vi "getDescription.vi"(8 "error in (no error)":errorcluster, 11 "Camera in":refnum<class "Camera.lvclass">) -> (0 "error out":errorcluster, 2 "description":T1={"serial"=4294967295, "type"=0, "sub_type"=0, "interface_type"=0, "bit_resolution"=0, "min_exposure_time_s"=nan, "max_exposure_time_s"=nan, "min_exposure_step_s"=nan, "min_delay_time_s"=nan, "max_delay_time_s"=nan, "min_delay_step_s"=nan, "min_width"=18446744073709551615, "min_height"=18446744073709551615, "max_width"=18446744073709551615, "max_height"=18446744073709551615, "roi_step_horz"=18446744073709551615, "roi_step_vert"=18446744073709551615, "roi_symmetric_horz"=FALSE, "roi_symmetric_vert"=FALSE, "has_timestamp_mode"=FALSE, "has_timestamp_mode_ascii_only"=FALSE, "pixelrate_vec"=[], "has_acquire_mode"=FALSE, "has_ext_acquire_mode"=FALSE, "has_metadata_mode"=FALSE, "has_ram"=FALSE, "binning_horz_vec"=[], "binning_vert_vec"=[]}, 3 "Camera out":refnum<class "Camera.lvclass">)   [LabVIEW 2020, in "Camera.lvclass"]
doc: "Gets the current configuration from the camera."
uses:
  Camera.lvclass
  Camera.lvclass/Camera.ctl
  CameraDescription.lvlib
  ImageSensor.lvlib
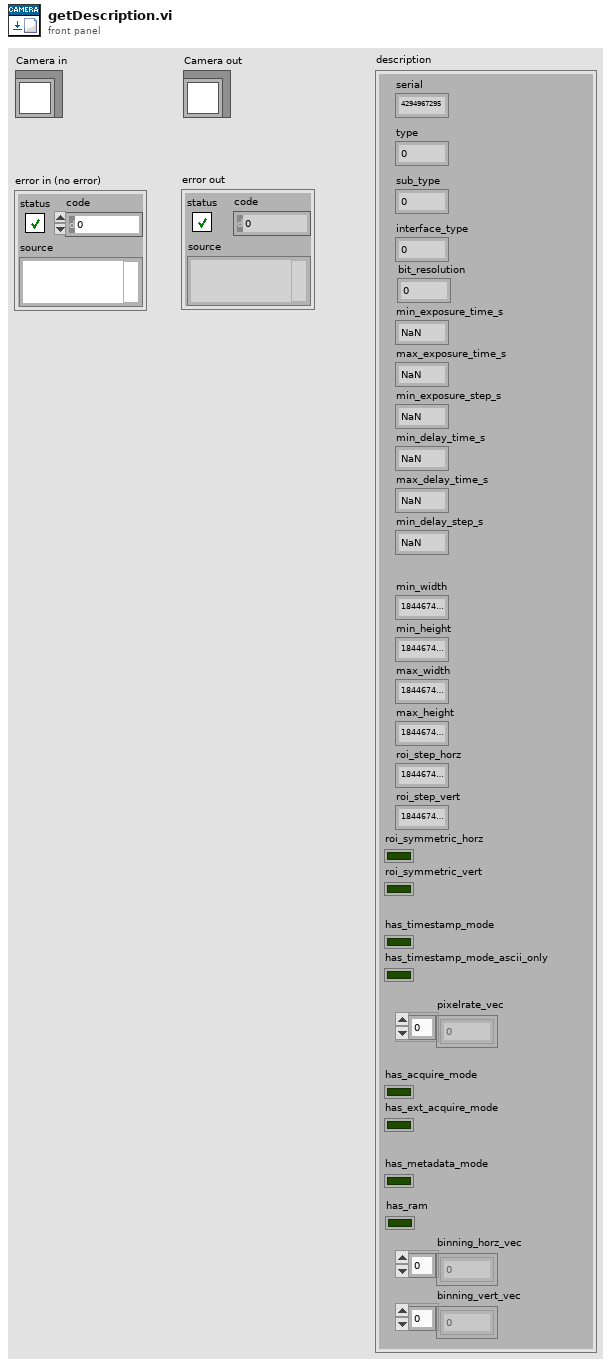
[diagram p1: front panel]
types:
  T1 = cluster{"serial":u32, "type":u16, "sub_type":u16, "interface_type":u16, "bit_resolution":u16, "min_exposure_time_s":dbl, "max_exposure_time_s":dbl, "min_exposure_step_s":dbl, "min_delay_time_s":dbl, "max_delay_time_s":dbl, "min_delay_step_s":dbl, "min_width":u64, "min_height":u64, "max_width":u64, "max_height":u64, "roi_step_horz":u64, "roi_step_vert":u64, "roi_symmetric_horz":bool, "roi_symmetric_vert":bool, "has_timestamp_mode":bool, "has_timestamp_mode_ascii_only":bool, "pixelrate_vec":u32[], "has_acquire_mode":bool, "has_ext_acquire_mode":bool, "has_metadata_mode":bool, "has_ram":bool, "binning_horz_vec":u16[], "binning_vert_vec":u16[]}
  T2 = cluster{"wSensorTypeDESC":u16, "wSensorSubTypeDESC":u16, "wMaxHorzResStdDESC":u16, "wMaxVertResStdDESC":u16, "wMaxHorzResExtDESC":u16, "wMaxVertResExtDESC":u16, "wDynResDESC":u16, "wMaxBinHorzDESC":u16, "wBinHorzSteppingDESC":u16, "wMaxBinVertDESC":u16, "wBinVertSteppingDESC":u16, "wRoiHorStepsDESC":u16, "wRoiVertStepsDESC":u16, "wNumADCsDESC":u16, "wMinSizeHorzDESC":u16, "dwPixelRateDESC":u32[], "wConvFactDESC":u16[], "sCoolingSetpoints":i16[], "wSoftRoiHorStepsDESC":u16, "wSoftRoiVertStepsDESC":u16, "wIRDESC":u16, "wMinSizeVertDESC":u16, "dwMinDelayDESC":u32, "dwMaxDelayDESC":u32, "dwMinDelayStepDESC":u32, "dwMinExposureDESC":u32, "dwMaxExposureDESC":u32, "dwMinExposureStepDESC":u32, "dwMinDelayIRDESC":u32, "dwMaxDelayIRDESC":u32, "dwMinExposureIRDESC":u32, "dwMaxExposureIRDESC":u32, "wTimeTableDESC":u16, "wDoubleImageDESC":u16, "sMinCoolSetDESC":i16, "sMaxCoolSetDESC":i16, "sDefaultCoolSetDESC":i16, "wPowerDownModeDESC":u16, "wOffsetRegulationDESC":u16, "wColorPatternDESC":u16, "wPatternTypeDESC":u16, "wNumCoolingSetpoints":u16, "dwGeneralCapsDESC1":u32, "dwGeneralCapsDESC2":u32, "dwExtSyncFrequency":u32[], "dwGeneralCapsDESC3":u32, "dwGeneralCapsDESC4":u32}
  T3 = cluster{"wDarkOffsetDESC3":u16, "dwGeneralCapsDESC3_1":u32, "dwGeneralCapsDESC3_2":u32, "dwGeneralCapsDESC3_3":u32, "dwGeneralCapsDESC3_4":u32, "wMinHorzResStdDESC3":u16, "wMinVertResStdDESC3":u16, "wMinHorzResExtDESC3":u16, "wMinVertResExtDESC3":u16, "dPixelsize_horzDESC3_um":dbl, "dPixelsize_vertDESC3_um":dbl, "dMinSensorTempWarningDESC3_C":dbl, "dMaxSensorTempWarningDESC3_C":dbl, "dMinCameraTempWarningDESC3_C":dbl, "dMaxCameraTempWarningDESC3_C":dbl, "dMinPowerTempWarningDESC3_C":dbl, "dMaxPowerTempWarningDESC3_C":dbl, "dMinPowerVoltageWarningDESC3_V":dbl, "dMaxPowerVoltageWarningDESC3_V":dbl, "dMinSensorTempErrorDESC3_C":dbl, "dMaxSensorTempErrorDESC3_C":dbl, "dMinCameraTempErrorDESC3_C":dbl, "dMaxCameraTempErrorDESC3_C":dbl, "dMinPowerTempErrorDESC3_C":dbl, "dMaxPowerTempErrorDESC3_C":dbl, "dMinPowerVoltageErrorDESC3_V":dbl, "dMaxPowerVoltageErrorDESC3_V":dbl}
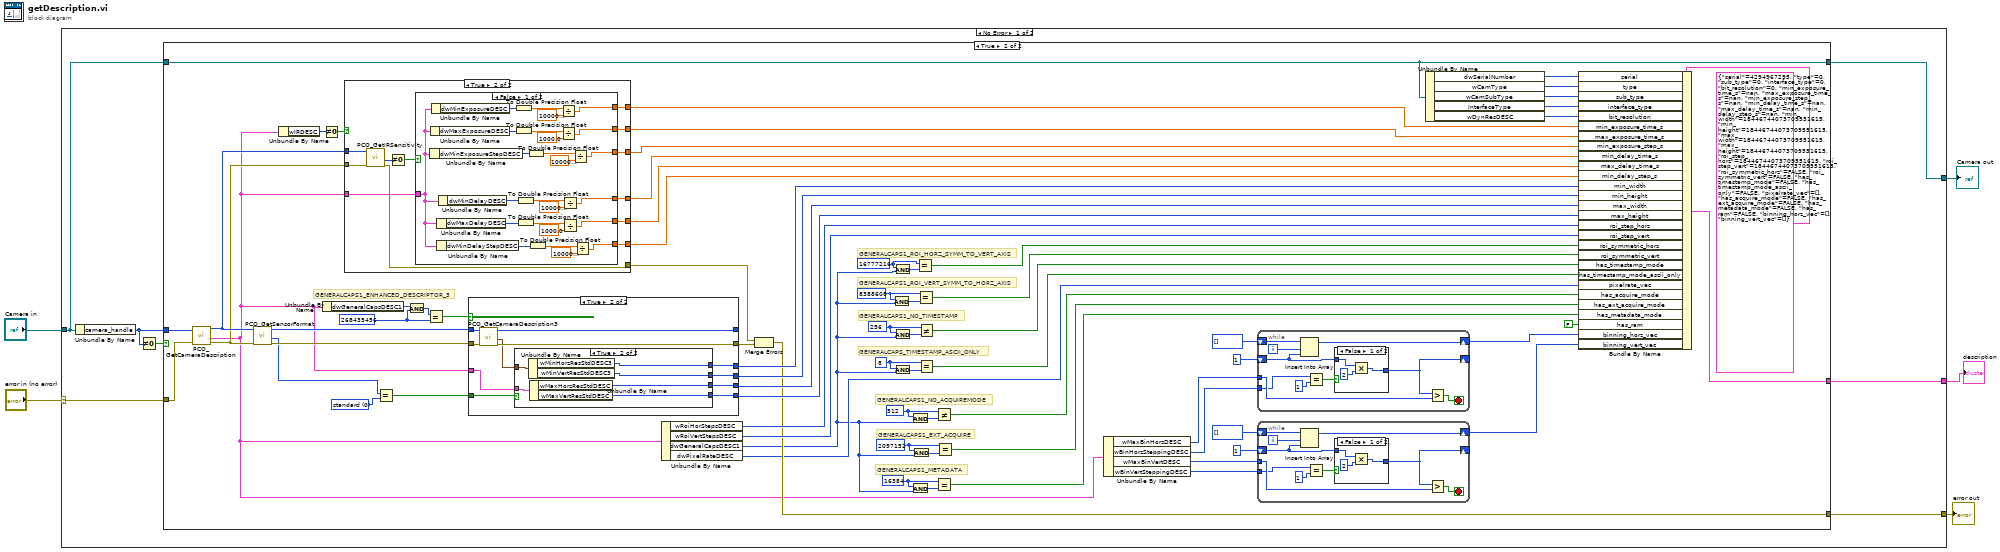
[diagram p0: block diagram]
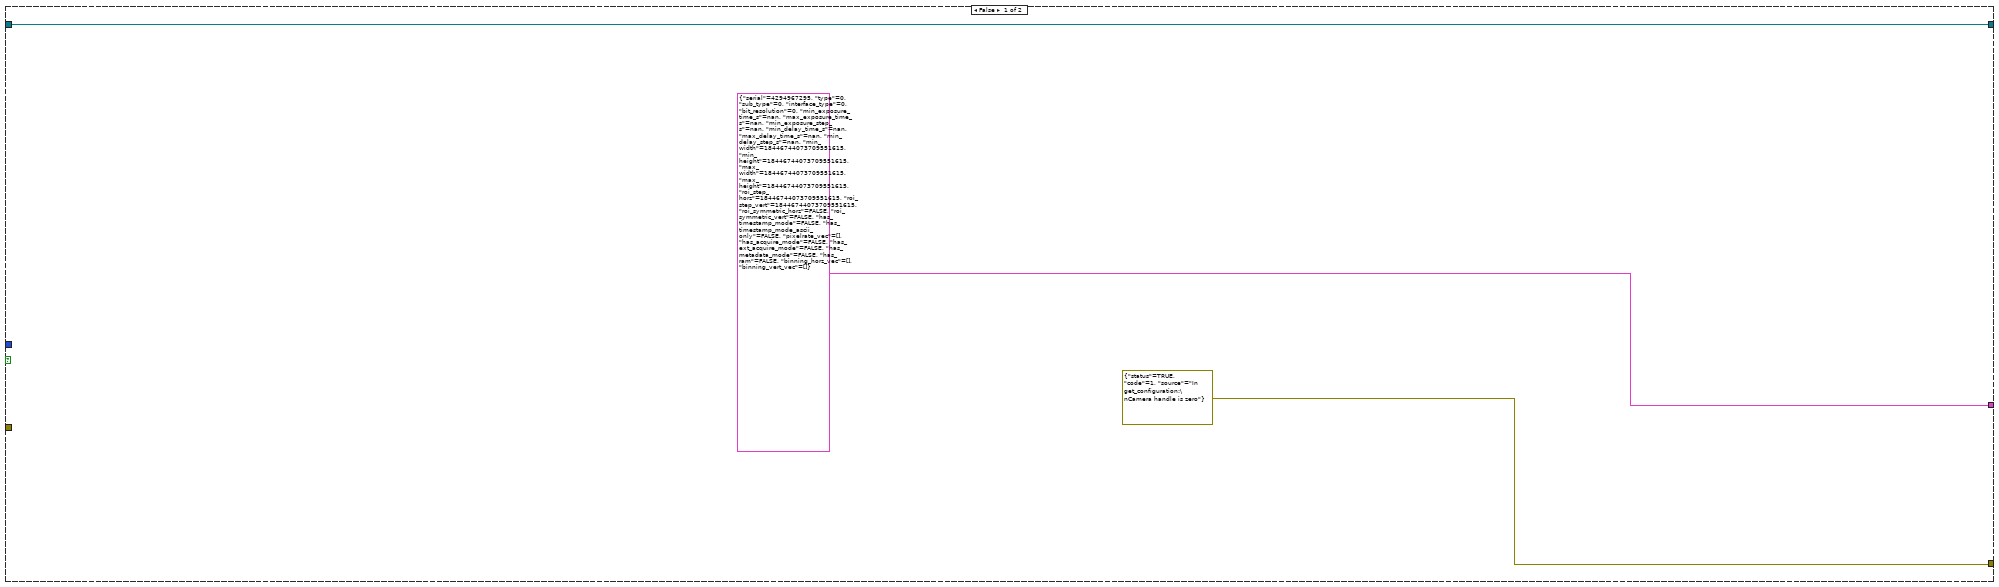
[diagram p2: hidden frame]
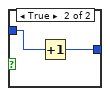
[diagram p3: hidden frame]
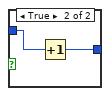
[diagram p4: hidden frame]
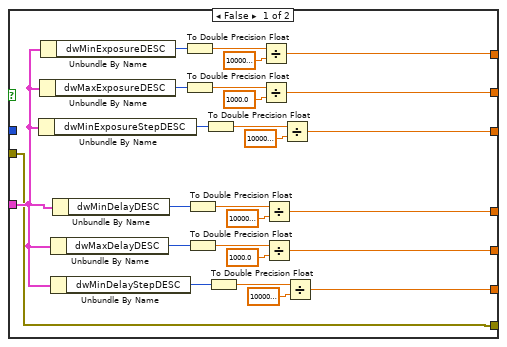
[diagram p5: hidden frame]
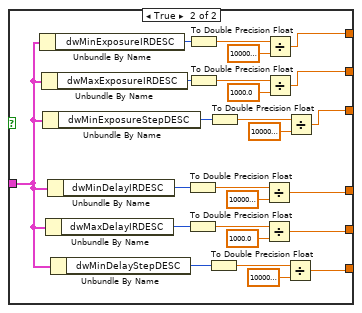
[diagram p6: hidden frame]
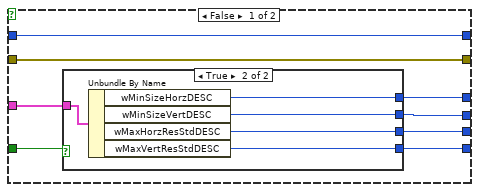
[diagram p7: hidden frame]
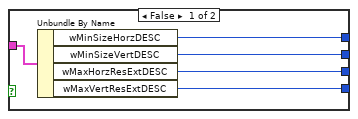
[diagram p8: hidden frame]
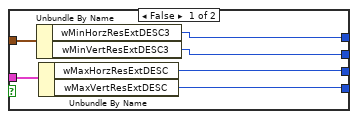
[diagram p9: hidden frame]
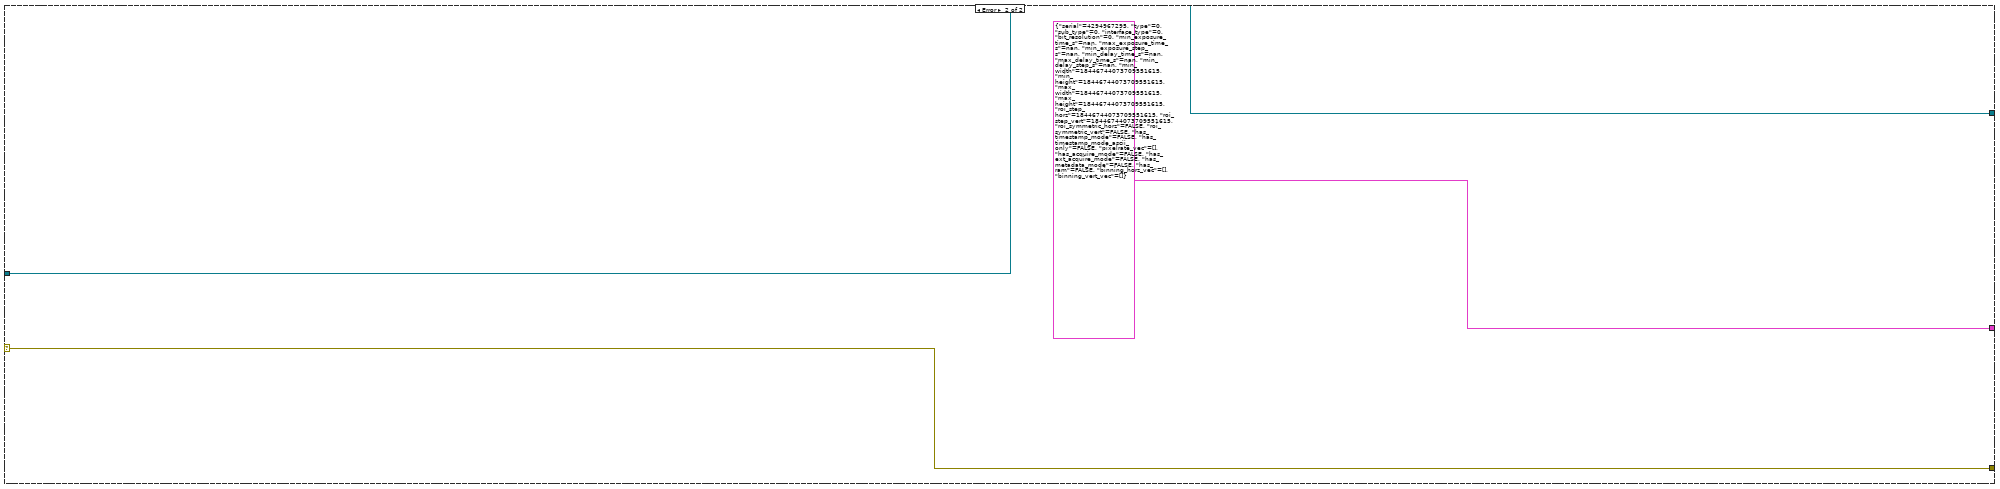
[diagram p10: hidden frame]
diagram:
  n1 = case shown="No Error" "error in (no error)" {
    selector: "error in (no error)" -> [w9 w250]
    tunnel: [w11 w250] -> w4
    tunnel: [w6 w249] -> w2
    tunnel: "Camera in" -> [w8 w249]
    tunnel: [w7 T1 {"serial"=4294967295, "type"=0, "sub_type"=0, "interface_type"=0, "bit_resolution"=0, "min_exposure_time_s"=nan, "max_exposure_time_s"=nan, "min_exposure_step_s"=nan, "min_delay_time_s"=nan, "max_delay_time_s"=nan, "min_delay_step_s"=nan, "min_width"=18446744073709551615, "min_height"=18446744073709551615, "max_width"=18446744073709551615, "max_height"=18446744073709551615, "roi_step_horz"=18446744073709551615, "roi_step_vert"=18446744073709551615, "roi_symmetric_horz"=FALSE, "roi_symmetric_vert"=FALSE, "has_timestamp_mode"=FALSE, "has_timestamp_mode_ascii_only"=FALSE, "pixelrate_vec"=[], "has_acquire_mode"=FALSE, "has_ext_acquire_mode"=FALSE, "has_metadata_mode"=FALSE, "has_ram"=FALSE, "binning_horz_vec"=[], "binning_vert_vec"=[]} ("description")] -> w1
    frame No Error {
      n2 = Unbundle By Name(w8) -> ("camera_handle"=w10:u64)
      n3 = Not Equal To 0?(x=w10) -> (x != 0?=w12:bool)
      n4 = case shown="True" w12 {
        tunnel: [errorcluster {"status"=TRUE, "code"=1, "source"="In get_configuration:\nCamera handle is zero"} ("error constant") w46] -> w11
        tunnel: w10 -> [_ w87]
        tunnel: w9 -> [_ w86]
        tunnel: w8 -> [w14 w25]
        tunnel: [T1 {"serial"=4294967295, "type"=0, "sub_type"=0, "interface_type"=0, "bit_resolution"=0, "min_exposure_time_s"=nan, "max_exposure_time_s"=nan, "min_exposure_step_s"=nan, "min_delay_time_s"=nan, "max_delay_time_s"=nan, "min_delay_step_s"=nan, "min_width"=18446744073709551615, "min_height"=18446744073709551615, "max_width"=18446744073709551615, "max_height"=18446744073709551615, "roi_step_horz"=18446744073709551615, "roi_step_vert"=18446744073709551615, "roi_symmetric_horz"=FALSE, "roi_symmetric_vert"=FALSE, "has_timestamp_mode"=FALSE, "has_timestamp_mode_ascii_only"=FALSE, "pixelrate_vec"=[], "has_acquire_mode"=FALSE, "has_ext_acquire_mode"=FALSE, "has_metadata_mode"=FALSE, "has_ram"=FALSE, "binning_horz_vec"=[], "binning_vert_vec"=[]} ("description") w88] -> w7
        tunnel: [w14 w25] -> w6
        frame False {
        }
        frame True {
          w38 = u32 16384 ("dwGeneralCapsDESC1")
          w40 = u32 2097152 ("dwGeneralCapsDESC1")
          w44 = u32 512 ("dwGeneralCapsDESC1")
          w50 = u32 8 ("dwGeneralCapsDESC1")
          w54 = u32 256 ("dwGeneralCapsDESC1")
          w59 = u32 8388608 ("dwGeneralCapsDESC1")
          w58 = u32 16777216 ("dwGeneralCapsDESC1")
          w79 = u16 0 items=["standard", "extended"] ("wSensor")
          w83 = u32 268435456 ("dwGeneralCapsDESC1")
          # "GENERALCAPS1_METADATA"
          # "GENERALCAPS1_EXT_ACQUIRE"
          # "GENERALCAPS1_NO_ACQUIREMODE"
          # "GENERALCAPS_TIMESTAMP_ASCII_ONLY"
          # "GENERALCAPS1_NO_TIMESTAMP"
          # "GENERALCAPS1_ROI_VERT_SYMM_TO_HORZ_AXIS"
          # "GENERALCAPS1_ROI_HORZ_SYMM_TO_VERT_AXIS"
          # "GENERALCAPS1_ENHANCED_DESCRIPTOR_3"
          n5 = call "PCO_GetCameraDescription.vi"("error in (no error)"=w86, "ph"=w87) -> ("error out"=w68:errorcluster, "strDescription"=w34:T2, "ph out"=w69:u64)  [unwired: 6 in, 1 out]
          n6 = call "PCO_GetSensorFormat.vi"("error in (no error)"=w68, "ph"=w69) -> ("error out"=w81:errorcluster, "wSensor"=w78:u16, "ph out"=w80:u64)  [unwired: 6 in, 1 out]
          n7 = Unbundle By Name(w34) -> ("wIRDESC"=w77:u16)
          n8 = Unbundle By Name(w34) -> ("dwGeneralCapsDESC1"=w85:u32)
          n9 = Not Equal To 0?(x=w77) -> (x != 0?=w76:bool)
          n10 = case shown="True" w76 {
            tunnel: w69 -> [_ w156]
            tunnel: w68 -> [w119 w155]
            tunnel: w34 -> [w125 w145]
            tunnel: [w141 w151] -> w75
            tunnel: [w124 w150] -> w74
            tunnel: [w123 w149] -> w73
            tunnel: [w122 w148] -> w72
            tunnel: [w121 w147] -> w71
            tunnel: [w120 w146] -> w70
            tunnel: [w119 w153] -> w48
            frame False {
              n11 = Unbundle By Name(w125) -> ("dwMinExposureStepDESC"=w135:u32)
              n12 = Unbundle By Name(w125) -> ("dwMaxExposureDESC"=w138:u32)
              n13 = Unbundle By Name(w125) -> ("dwMinExposureDESC"=w144:u32)
              n14 = Unbundle By Name(w125) -> ("dwMaxDelayDESC"=w129:u32)
              n15 = Unbundle By Name(w125) -> ("dwMinDelayStepDESC"=w126:u32)
              n16 = Unbundle By Name(w125) -> ("dwMinDelayDESC"=w134:u32)
              n17 = To Double Precision Float(number=w144) -> (double precision float=w143:dbl)
              n18 = To Double Precision Float(number=w138) -> (double precision float=w140:dbl)
              n19 = To Double Precision Float(number=w134) -> (double precision float=w133:dbl)
              n20 = To Double Precision Float(number=w129) -> (double precision float=w131:dbl)
              n21 = To Double Precision Float(number=w135) -> (double precision float=w137:dbl)
              n22 = To Double Precision Float(number=w126) -> (double precision float=w128:dbl)
              n23 = Divide(x=w143, y=1000000000.0) -> (x/y=w141:dbl)
              n24 = Divide(x=w140, y=1000.0) -> (x/y=w124:dbl)
              n25 = Divide(x=w133, y=1000000000.0) -> (x/y=w122:dbl)
              n26 = Divide(x=w131, y=1000.0) -> (x/y=w121:dbl)
              n27 = Divide(x=w137, y=1000000000.0) -> (x/y=w123:dbl)
              n28 = Divide(x=w128, y=1000000000.0) -> (x/y=w120:dbl)
            }
            frame True {
              n29 = call "PCO_GetIRSensitivity.vi"("error in (no error)"=w155, "ph"=w156) -> ("error out"=w153:errorcluster, "wIR"=w154:u16)  [unwired: 6 in, 2 out]
              n30 = Not Equal To 0?(x=w154) -> (x != 0?=w152:bool)
              n31 = case shown="False" w152 {
                tunnel: [w169 w193] -> w151
                tunnel: [w168 w192] -> w150
                tunnel: [w167 w191] -> w149
                tunnel: [w166 w190] -> w148
                tunnel: [w165 w189] -> w147
                tunnel: [w164 w188] -> w146
                tunnel: w145 -> [w157 w194]
                frame False {
                  n32 = Unbundle By Name(w157) -> ("dwMinExposureStepDESC"=w176:u32)
                  n33 = Unbundle By Name(w157) -> ("dwMaxExposureDESC"=w178:u32)
                  n34 = Unbundle By Name(w157) -> ("dwMinExposureDESC"=w181:u32)
                  n35 = Unbundle By Name(w157) -> ("dwMaxDelayDESC"=w172:u32)
                  n36 = Unbundle By Name(w157) -> ("dwMinDelayStepDESC"=w170:u32)
                  n37 = Unbundle By Name(w157) -> ("dwMinDelayDESC"=w175:u32)
                  n38 = To Double Precision Float(number=w181) -> (double precision float=w180:dbl)
                  n39 = To Double Precision Float(number=w178) -> (double precision float=w179:dbl)
                  n40 = To Double Precision Float(number=w175) -> (double precision float=w174:dbl)
                  n41 = To Double Precision Float(number=w172) -> (double precision float=w173:dbl)
                  n42 = To Double Precision Float(number=w176) -> (double precision float=w177:dbl)
                  n43 = To Double Precision Float(number=w170) -> (double precision float=w171:dbl)
                  n44 = Divide(x=w180, y=1000000000.0) -> (x/y=w169:dbl)
                  n45 = Divide(x=w179, y=1000.0) -> (x/y=w168:dbl)
                  n46 = Divide(x=w174, y=1000000000.0) -> (x/y=w166:dbl)
                  n47 = Divide(x=w173, y=1000.0) -> (x/y=w165:dbl)
                  n48 = Divide(x=w177, y=1000000000.0) -> (x/y=w167:dbl)
                  n49 = Divide(x=w171, y=1000000000.0) -> (x/y=w164:dbl)
                }
                frame True {
                  n50 = Unbundle By Name(w194) -> ("dwMinExposureIRDESC"=w206:u32)
                  n51 = Unbundle By Name(w194) -> ("dwMaxExposureIRDESC"=w203:u32)
                  n52 = Unbundle By Name(w194) -> ("dwMinExposureStepDESC"=w201:u32)
                  n53 = Unbundle By Name(w194) -> ("dwMaxDelayIRDESC"=w197:u32)
                  n54 = Unbundle By Name(w194) -> ("dwMinDelayIRDESC"=w200:u32)
                  n55 = Unbundle By Name(w194) -> ("dwMinDelayStepDESC"=w195:u32)
                  n56 = To Double Precision Float(number=w200) -> (double precision float=w199:dbl)
                  n57 = To Double Precision Float(number=w197) -> (double precision float=w198:dbl)
                  n58 = To Double Precision Float(number=w206) -> (double precision float=w205:dbl)
                  n59 = To Double Precision Float(number=w203) -> (double precision float=w204:dbl)
                  n60 = To Double Precision Float(number=w195) -> (double precision float=w196:dbl)
                  n61 = To Double Precision Float(number=w201) -> (double precision float=w202:dbl)
                  n62 = Divide(x=w199, y=1000000000.0) -> (x/y=w190:dbl)
                  n63 = Divide(x=w198, y=1000.0) -> (x/y=w189:dbl)
                  n64 = Divide(x=w205, y=1000000000.0) -> (x/y=w193:dbl)
                  n65 = Divide(x=w204, y=1000.0) -> (x/y=w192:dbl)
                  n66 = Divide(x=w196, y=1000000000.0) -> (x/y=w188:dbl)
                  n67 = Divide(x=w202, y=1000000000.0) -> (x/y=w191:dbl)
                }
              }
            }
          }
          n68 = Equal?(x=w78, y=w79) -> (x = y?=w67:bool)
          n69 = And(x=w85, y=w83) -> (x .and. y?=w84:u32)
          n70 = Equal?(x=w84, y=w83) -> (x = y?=w82:bool)
          n71 = case shown="True" w82 {
            tunnel: w81 -> [w214 w235]
            tunnel: w80 -> [w213 w234]
            tunnel: w34 -> [w211 w230]
            tunnel: [w214 w232] -> w47
            tunnel: [w213 w233] -> _
            tunnel: w67 -> [w212 w231]
            tunnel: [w210 w228] -> w66
            tunnel: [w209 w227] -> w65
            tunnel: [w208 w226] -> w64
            tunnel: [w207 w225] -> w63
            frame False {
              n72 = case shown="True" w212 {
                tunnel: w211 -> [w219 w224]
                tunnel: [w215 w223] -> w210
                tunnel: [w216 w222] -> w209
                tunnel: [w217 w221] -> w208
                tunnel: [w218 w220] -> w207
                frame False {
                  n73 = Unbundle By Name(w219) -> ("wMinSizeHorzDESC"=w215:u16, "wMinSizeVertDESC"=w216:u16, "wMaxHorzResExtDESC"=w217:u16, "wMaxVertResExtDESC"=w218:u16)
                }
                frame True {
                  n74 = Unbundle By Name(w224) -> ("wMinSizeHorzDESC"=w223:u16, "wMinSizeVertDESC"=w222:u16, "wMaxHorzResStdDESC"=w221:u16, "wMaxVertResStdDESC"=w220:u16)
                }
              }
            }
            frame True {
              n75 = call "PCO_GetCameraDescription3.vi"("error in (no error)"=w235, "ph"=w234) -> ("error out"=w232:errorcluster, "strDescription"=w229:T3, "ph out"=w233:u64)  [unwired: 6 in, 1 out]
              n76 = case shown="True" w231 {
                tunnel: w230 -> [w240 w247]
                tunnel: [w236 w243] -> w228
                tunnel: [w237 w242] -> w227
                tunnel: [w238 w246] -> w226
                tunnel: [w239 w245] -> w225
                tunnel: w229 -> [w241 w244]
                frame False {
                  n77 = Unbundle By Name(w241) -> ("wMinHorzResExtDESC3"=w236:u16, "wMinVertResExtDESC3"=w237:u16)
                  n78 = Unbundle By Name(w240) -> ("wMaxHorzResExtDESC"=w238:u16, "wMaxVertResExtDESC"=w239:u16)
                }
                frame True {
                  n79 = Unbundle By Name(w244) -> ("wMinHorzResStdDESC3"=w243:u16, "wMinVertResStdDESC3"=w242:u16)
                  n80 = Unbundle By Name(w247) -> ("wMaxHorzResStdDESC"=w246:u16, "wMaxVertResStdDESC"=w245:u16)
                }
              }
            }
          }
          n81 = Unbundle By Name(w34) -> ("wRoiHorStepsDESC"=w62:u16, "wRoiVertStepsDESC"=w61:u16, "dwGeneralCapsDESC1"=w36:u32, "dwPixelRateDESC"=w45:u32[])
          n82 = Merge Errors(w48, w47) -> (w46:errorcluster)
          n83 = And(x=w59, y=w36) -> (x .and. y?=w60:u32)
          n84 = And(x=w58, y=w36) -> (x .and. y?=w57:u32)
          n85 = And(x=w54, y=w36) -> (x .and. y?=w53:u32)
          n86 = And(x=w50, y=w36) -> (x .and. y?=w51:u32)
          n87 = And(x=w44, y=w36) -> (x .and. y?=w43:u32)
          n88 = And(x=w38, y=w36) -> (x .and. y?=w37:u32)
          n89 = And(x=w40, y=w36) -> (x .and. y?=w41:u32)
          n90 = Equal?(x=w58, y=w57) -> (x = y?=w56:bool)
          n91 = Equal?(x=w59, y=w60) -> (x = y?=w55:bool)
          n92 = Not Equal?(x=w54, y=w53) -> (x != y?=w52:bool)
          n93 = Equal?(x=w50, y=w51) -> (x = y?=w49:bool)
          n94 = Not Equal?(x=w44, y=w43) -> (x != y?=w42:bool)
          n95 = Equal?(x=w38, y=w37) -> (x = y?=w35:bool)
          n96 = Equal?(x=w40, y=w41) -> (x = y?=w39:bool)
          n97 = Unbundle By Name(w34) -> ("wMaxBinHorzDESC"=w33:u16, "wBinHorzSteppingDESC"=w32:u16, "wMaxBinVertDESC"=w27:u16, "wBinVertSteppingDESC"=w26:u16)
          n98 = while {
            tunnel: w33 -> [w109]
            tunnel: w32 -> [w108]
            shift-right: [w111] -> w23
            shift-left: u16[] [] ("binning_horz_vec") -> [w113]
            shift-right: [w104] -> _
            shift-left: u16 1 -> [w105]
            i -> [w112]
            stop <- w110 stop-if-true
            n99 = Insert Into Array(array=w113, index=w112, new element=w105) -> (w111:u16[])
            n100 = Equal?(x=w108, y=u16 1 ("wBinHorzSteppingDESC")) -> (x = y?=w106:bool)
            n101 = case shown="False" w106 {
              tunnel: w105 -> [w115 w118]
              tunnel: [w116 w117] -> w104
              frame False {
                n102 = Multiply(x=w115, y=u16 2) -> (x*y=w116:u16)
              }
              frame True {
                n103 = Increment(x=w118) -> (x+1=w117:u16)
              }
            }
            n104 = Greater?(x=w104, y=w109) -> (0:w110:bool)
          }
          n105 = while {
            tunnel: w27 -> [w94]
            tunnel: w26 -> [w93]
            shift-right: [w96] -> w22
            shift-left: u16[] [] ("binning_horz_vec") -> [w98]
            shift-right: [w89] -> _
            shift-left: u16 1 -> [w90]
            i -> [w97]
            stop <- w95 stop-if-true
            n106 = Insert Into Array(array=w98, index=w97, new element=w90) -> (w96:u16[])
            n107 = Equal?(x=w93, y=u16 1 ("wBinHorzSteppingDESC")) -> (x = y?=w91:bool)
            n108 = case shown="False" w91 {
              tunnel: w90 -> [w100 w103]
              tunnel: [w101 w102] -> w89
              frame False {
                n109 = Multiply(x=w100, y=u16 2) -> (x*y=w101:u16)
              }
              frame True {
                n110 = Increment(x=w103) -> (x+1=w102:u16)
              }
            }
            n111 = Greater?(x=w89, y=w94) -> (0:w95:bool)
          }
          n112 = Unbundle By Name(w25) -> ("dwSerialNumber"=w21:u32, "wCamType"=w20:u16, "wCamSubType"=w19:u16, "InterfaceType"=w18:u16, "wDynResDESC"=w17:u16)
          n113 = Bundle By Name(cluster=T1 {"serial"=4294967295, "type"=0, "sub_type"=0, "interface_type"=0, "bit_resolution"=0, "min_exposure_time_s"=nan, "max_exposure_time_s"=nan, "min_exposure_step_s"=nan, "min_delay_time_s"=nan, "max_delay_time_s"=nan, "min_delay_step_s"=nan, "min_width"=18446744073709551615, "min_height"=18446744073709551615, "max_width"=18446744073709551615, "max_height"=18446744073709551615, "roi_step_horz"=18446744073709551615, "roi_step_vert"=18446744073709551615, "roi_symmetric_horz"=FALSE, "roi_symmetric_vert"=FALSE, "has_timestamp_mode"=FALSE, "has_timestamp_mode_ascii_only"=FALSE, "pixelrate_vec"=[], "has_acquire_mode"=FALSE, "has_ext_acquire_mode"=FALSE, "has_metadata_mode"=FALSE, "has_ram"=FALSE, "binning_horz_vec"=[], "binning_vert_vec"=[]} ("description"), "serial"=w21, "type"=w20, "sub_type"=w19, "interface_type"=w18, "bit_resolution"=w17, "min_exposure_time_s"=w75, "max_exposure_time_s"=w74, "min_exposure_step_s"=w73, "min_delay_time_s"=w72, "max_delay_time_s"=w71, "min_delay_step_s"=w70, "min_width"=w66, "min_height"=w65, "max_width"=w64, "max_height"=w63, "roi_step_horz"=w62, "roi_step_vert"=w61, "roi_symmetric_horz"=w56, "roi_symmetric_vert"=w55, "has_timestamp_mode"=w52, "has_timestamp_mode_ascii_only"=w49, "pixelrate_vec"=w45, "has_acquire_mode"=w42, "has_ext_acquire_mode"=w39, "has_metadata_mode"=w35, "has_ram"=FALSE, "binning_horz_vec"=w23, "binning_vert_vec"=w22) -> (w88:T1)
        }
      }
    }
    frame Error {
    }
  }
  "error out" <- w4
  "Camera out" <- w2
  "description" <- w1
